vi "方程子VI2.vi"   [LabVIEW 2018]
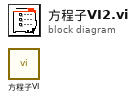
[diagram p0: block diagram]
diagram:
  n1 = call "方程子VI.vi"() -> ()  [unwired: 12 in]
